vi "run_embedding.vi"(0 "llm_openai_embedding in":refnum<class "llm_openai_embedding.lvclass">, 5 "data":refnum<class "abstract_message_base.lvclass">[](array[class]), 11 "error in (no error)":errorcluster) -> (4 "llm_openai_embedding out":refnum<class "llm_openai_embedding.lvclass">, 6 "embedding response":refnum<class "message_vectors.lvclass">[](array[class]), 15 "error out":errorcluster)   [LabVIEW 2020, in "llm_openai_embedding.lvclass"]
uses:
  llm_openai_embedding.lvclass
  abstract_message_base/abstract_message_base.lvclass
  message_vectors/message_vectors.lvclass
  <vilib>/httpClient/POSTBuffer.vi
  llm_openai_embedding.lvclass/llm_openai_embedding.ctl
  <vilib>/httpClient/LabVIEWHTTPClient.lvlib
panel:
  out "body":string
  out "headers":string
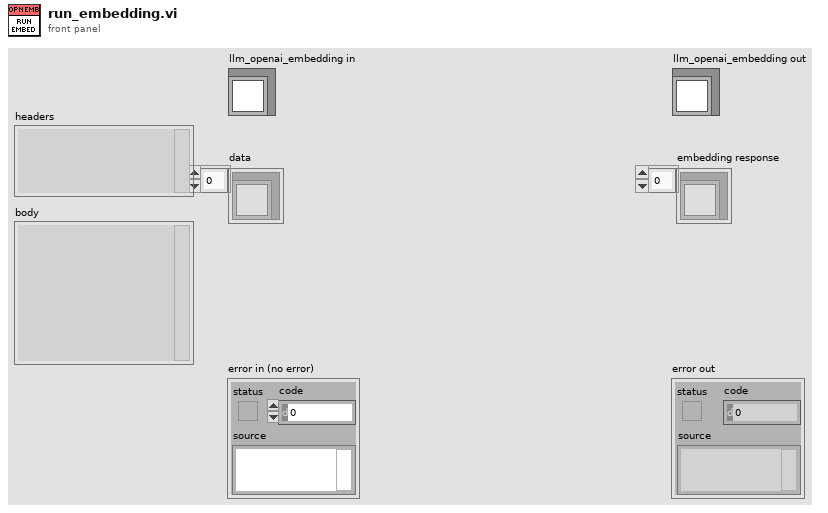
[diagram p1: front panel]
types:
  T1 = typedef "LabVIEWHTTPClient.lvlib/ClientHandle.ctl" = refnum<k1>
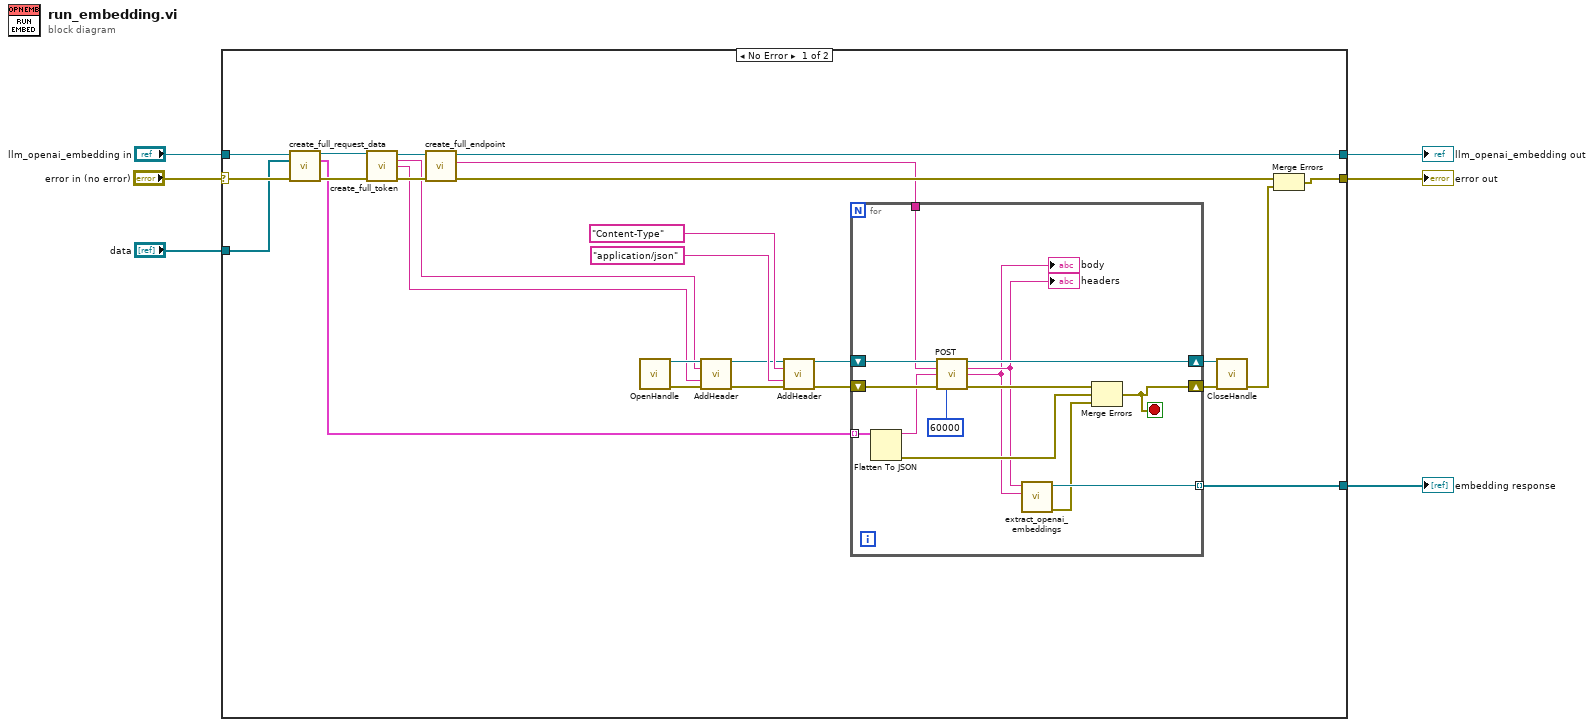
[diagram p0: block diagram]
diagram:
  n1 = case shown="No Error" "error in (no error)" {
    selector: "error in (no error)" -> [w13 w48]
    tunnel: [w9 w48] -> w5
    tunnel: [w21 w47] -> w4
    tunnel: "llm_openai_embedding in" -> [w14 w47]
    tunnel: "data" -> [w12 _]
    tunnel: [w7 _] -> w1
    frame No Error {
      n2 = call-dynamic "create_full_request_data.vi"("llm_openai_embedding in"=w14, "data"=w12, "error in (no error)"=w13) -> ("llm_openai_embedding out"=w15:refnum<class "llm_openai_embedding.lvclass">, "request_data"=w11:cluster{"input":string, "model":string}[], "error out"=w16:errorcluster)  [unwired: 10 in]
      n3 = call-dynamic "create_full_token.vi"("llm_openai_embedding in"=w15, "error in (no error)"=w16) -> ("llm_openai_embedding out"=w22:refnum<class "llm_openai_embedding.lvclass">, "header"=w18:string, "token"=w17:string, "error out"=w23:errorcluster)  [unwired: 10 in]
      n4 = call-dynamic "create_full_endpoint.vi"("error in (no error)"=w23, "llm_openai_embedding in"=w22) -> ("error out"=w20:errorcluster, "endpoint"=w19:string, "llm_openai_embedding out"=w21:refnum<class "llm_openai_embedding.lvclass">)  [unwired: 7 in]
      n5 = call <vilib>:"OpenHandle.vi"() -> ("client handle out"=w32:T1, "error out"=w31:errorcluster)  [unwired: 14 in]
      n6 = call <vilib>:"AddHeader.vi"("client handle"=w32, "header"=w18, "value"=w17, "error in (no error)"=w31) -> ("client handle out"=w28:T1, "error out"=w26:errorcluster)  [unwired: 10 in]
      n7 = call <vilib>:"AddHeader.vi"("client handle"=w28, "header"="Content-Type", "value"="application/json", "error in (no error)"=w26) -> ("client handle out"=w27:T1, "error out"=w25:errorcluster)  [unwired: 10 in]
      n8 = for {
        tunnel: w19 -> [w42]
        shift-right: [w44] -> w24
        shift-left: w27 -> [w46]
        tunnel: w11 -> [w40] mode=indexing
        shift-right: [w37] -> w10
        shift-left: w25 -> [w45]
        tunnel: [w34] -> w7 mode=indexing
        stop <- w37 stop-if-true
        n9 = Flatten To JSON(anything=w40) -> (JSON string=w39:string, 11:w38:errorcluster)  [unwired: 2 in]
        n10 = call-poly <vilib>:"POST.vi"("client handle"=w46, "url"=w42, "buffer"=w39, "error in (no error)"=w45, "timeout (10000)"=60000) -> ("client handle out"=w44:T1, "headers"=w36:string, "body"=w35:string, "error out"=w41:errorcluster)  [unwired: 7 in]
        "headers" <- w36
        "body" <- w35
        n11 = call "extract_openai_embeddings.vi"("body"=w35, "headers"=w36) -> ("error out"=w33:errorcluster, "vector response"=w34:refnum<class "message_vectors.lvclass">)  [unwired: 8 in]
        n12 = Merge Errors(w41, w38, w33) -> (w37:errorcluster)
      }
      n13 = call <vilib>:"CloseHandle.vi"("client handle"=w24, "error in (no error)"=w10) -> ("error out"=w8:errorcluster)  [unwired: 13 in]
      n14 = Merge Errors(w20, w8) -> (w9:errorcluster)
    }
    frame Error {
    }
  }
  "error out" <- w5
  "llm_openai_embedding out" <- w4
  "embedding response" <- w1
